vi "Touchpad_1ChLoadCell9237.vi"() -> ()   [LabVIEW 2013]
uses:
  <vilib>/Utility/error.llb/DialogType.ctl
  <vilib>/DAQmx/configure/timing.llb/DAQmx Timing (Sample Clock).vi
  <vilib>/DAQmx/read.llb/DAQmx Read (Analog Wfm 1Chan NSamp).vi
panel:
  in  "Samples/ch":i32=100000
  out "Waveform Chart":waveform(dbl)(graph)
  in  "Sample Mode":i32(ring)=10123 items=["Finite Samples"=10178, "Continuous Samples"=10123, "Hardware Timed Single Point"=12522]
  in  "File Record Name":path=path "D:/LHI/Pengujian/2026/Touchpad_Impact_Piezo/Data/1ChLoadCell9237_1ChImpact6008/testsinyal_9237_formasi_1_00.txt" caption="Filename"
  in  "DAQ Channel":refnum<k21>="LC_SBeam_100N_cDaq9237"
  in  "Rate (Hz)":dbl=2000.0 format="%0.2f"
  in  "stop":bool
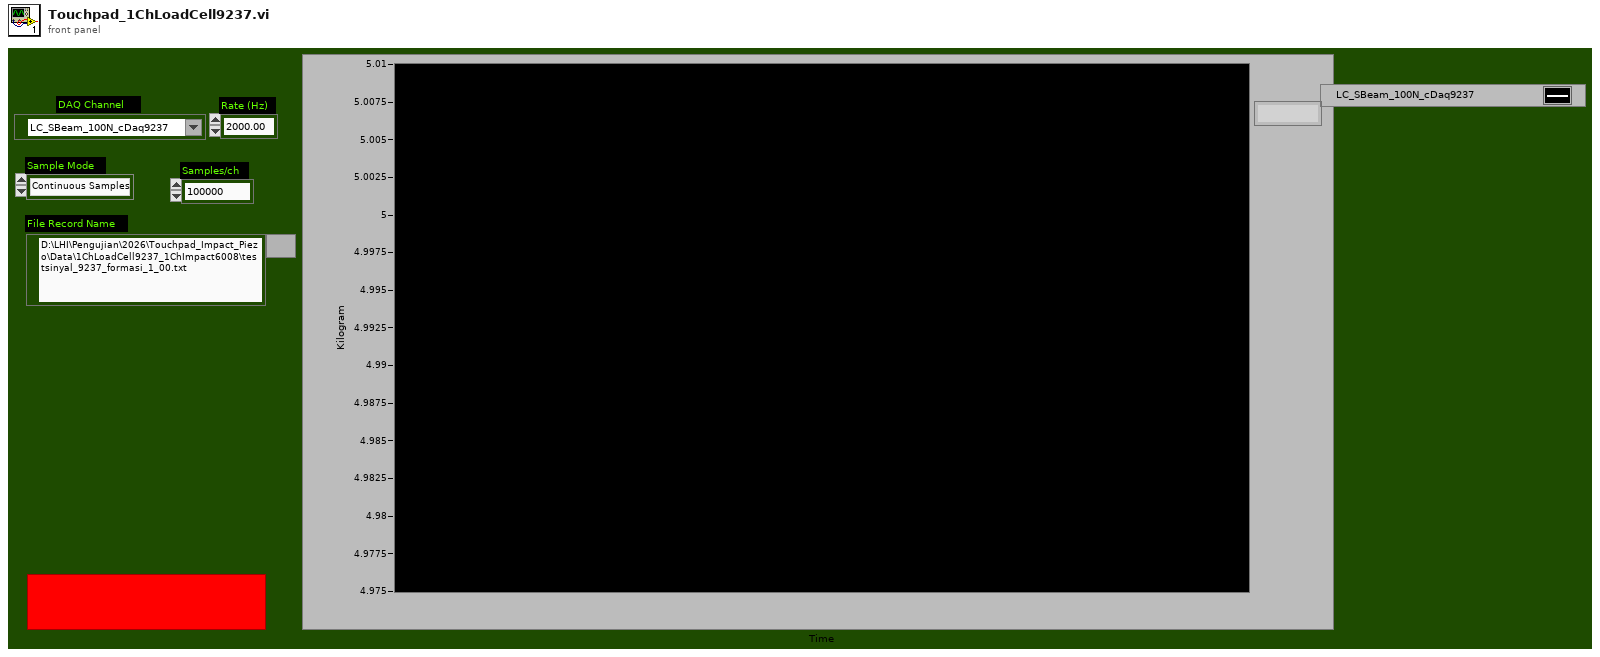
[diagram p1: front panel]
types:
  T1 = typedef "DialogType.ctl" = u16
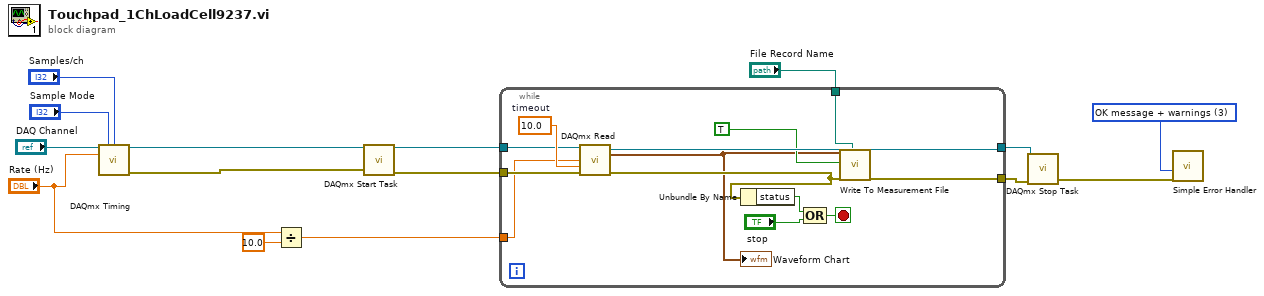
[diagram p0: block diagram]
diagram:
  w14 = T1 3 items=["no dialog", "OK message", "continue or stop message", "OK message + warnings", "continue/stop + warnings"] ("type of dialog (OK msg:1)")
  n1 = call-poly <vilib>:"DAQmx Timing.vi"("task/channels in"="DAQ Channel", "sample mode"="Sample Mode", "samples per channel"="Samples/ch", "rate"="Rate (Hz)") -> ("task out"=w5:refnum<k21>, "error out"=w4:errorcluster)  [unwired: 10 in]
  n2 = Divide(x="Rate (Hz)", y=10.0) -> (x/y=w6:dbl)
  n3 = call <vilib>:"DAQmx Start Task.vi"("task/channels in"=w5, "error in"=w4) -> ("task out"=w3:refnum<k21>, "error out"=w2:errorcluster)  [unwired: 12 in]
  n4 = while {
    tunnel: w2 -> [w27]
    tunnel: w3 -> [w26]
    tunnel: [w21] -> w13
    tunnel: [w23] -> w12
    tunnel: "File Record Name" -> [w18]
    tunnel: w6 -> [w16]
    stop <- w24 stop-if-true
    w28 = 10.0  # timeout
    n5 = call-poly <vilib>:"DAQmx Read.vi"("task/channels in"=w26, "number of samples per channel"=w16, "timeout"=w28, "error in"=w27) -> ("task out"=w23:refnum<k21>, "data"=w17:waveform(dbl), "error out"=w22:errorcluster)  [unwired: 9 in]
    "Waveform Chart" <- w17
    n6 = Unbundle By Name(w22) -> ("status"=w25:bool)
    n7 = Compound Arithmetic op=OR(w25, "stop") -> (w24:bool)
    n8 = call "Write To Measurement File"("Signals"=w17, "Enable"=TRUE ("Enable Rekam"), "error in (no error)"=w22, "Filename"=w18) -> ("error out"=w21:errorcluster)  [unwired: 13 in, 2 out]
  }
  n9 = call <vilib>:"DAQmx Stop Task.vi"("task/channels in"=w12, "error in"=w13) -> ("error out"=w1:errorcluster)  [unwired: 12 in, 1 out]
  n10 = call <vilib>:"Simple Error Handler.vi"("type of dialog (OK msg:1)"=w14, "error in (no error)"=w1) -> ()  [unwired: 3 in, 5 out]
